vi "SetAxisParameter.vi"(8 "error in (no error)":errorcluster, 11 "DMC 3600 in":refnum<class "DMC 3600.lvclass">) -> (0 "error out":errorcluster, 3 "DMC 3600 out":refnum<class "DMC 3600.lvclass">)   [LabVIEW 2019, in "DMC 3600.lvclass"]
uses:
  DMC 3600.lvclass
  LLB/DMC3600/LTDMC.lvlib
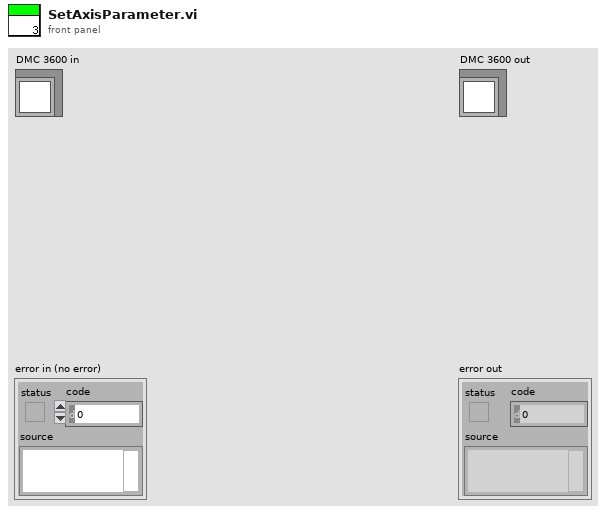
[diagram p1: front panel]
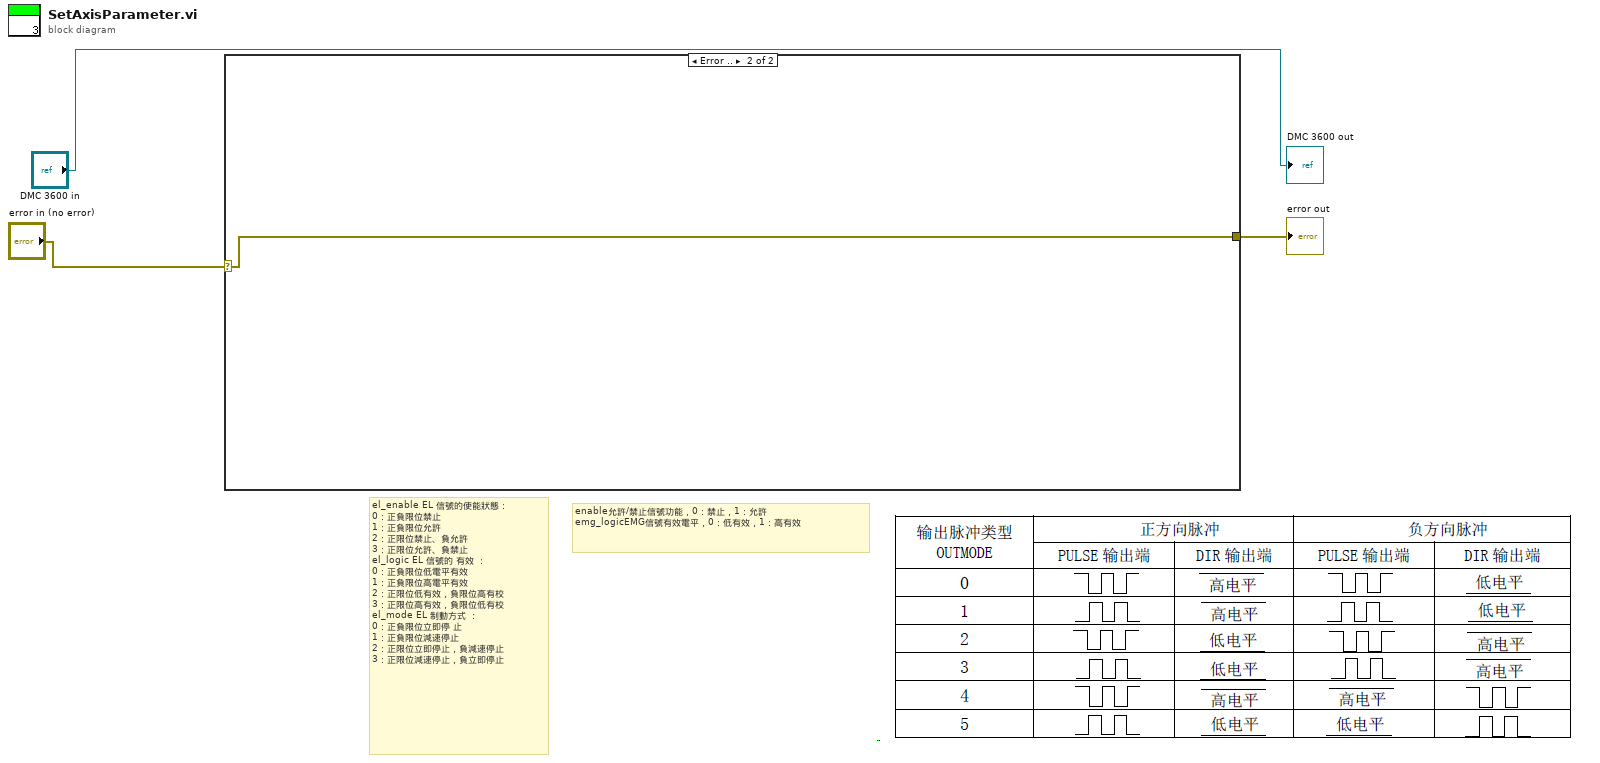
[diagram p0: block diagram]
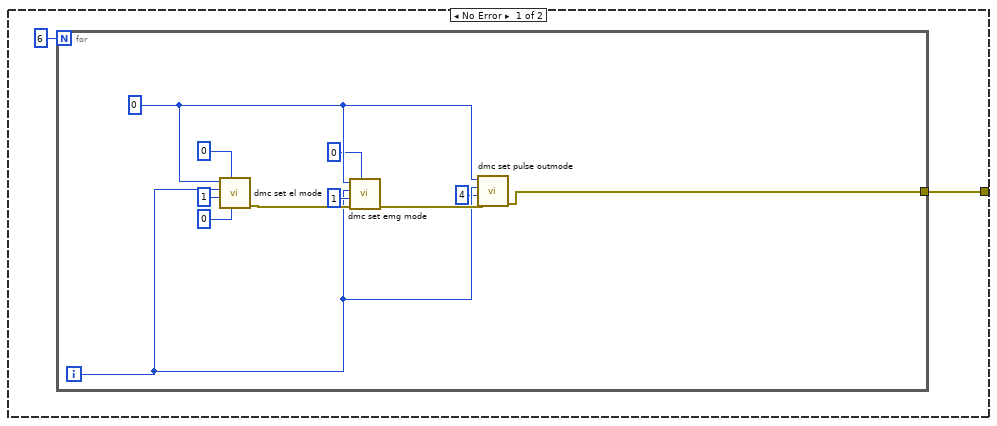
[diagram p2: hidden frame]
diagram:
  # "enable允許/禁止信號功能，0：禁止，1：允許\nemg_logicEMG信號有效電平，0：低有效，1：高有效"
  # "el_enable EL 信號的使能狀態：\n0：正負限位禁止\n1：正負限位允許\n2：正限位禁止、負允許\n3：正限位允許、負禁止\nel_logic EL 信號的 有效 ：\n0：正負限位低電平有效\n1：正負限位高電平有效\n2：正限位低有效，負限位高有校\n3：正限位高有效，負限位低有校\nel_mode EL 制動方式 ：\n0：正負限位立即停 止\n1：正負限位減速停止\n2：正限位立即停止，負減速停止\n3：正限位減速停止，負立即停止"
  n1 = case shown="Error .." "error in (no error)" {
    selector: "error in (no error)" -> [_ w17]
    tunnel: [w4 w17] -> w1
    frame No Error {
      n2 = for {
        N: 6 -> [_]
        tunnel: [w6] -> w4
        i -> [w8]
        w16 = u16 0 ("CardNo")
        n3 = call "dmc set el mode.vi"("el_mode"=u16 0, "el_logic"=u16 0, "enable"=u16 1, "axis"=w8, "CardNo"=w16) -> ("error out"=w12:errorcluster)  [unwired: 5 in, 1 out]
        n4 = call "dmc set emg mode.vi"("emg_logic"=u16 0, "error in (no error)"=w12, "enable"=u16 1, "axis"=w8, "CardNo"=w16) -> ("error out"=w9:errorcluster)  [unwired: 5 in, 1 out]
        n5 = call "dmc set pulse outmode.vi"("error in (no error)"=w9, "outmode"=u16 4, "axis"=w8, "CardNo"=w16) -> ("error out"=w6:errorcluster)  [unwired: 6 in, 1 out]
      }
    }
    frame Error {
    }
  }
  "error out" <- w1
  "DMC 3600 out" <- "DMC 3600 in"
